vi "Izhikevich_model.vi"() -> ()   [LabVIEW 2019]
panel:
  in  "Array":dbl[](array[slide]) scale=0.0..15.0
  out "u":T1(graph)
  in  "Address Selector":i32[](array[numeric])
  out "v":T1(graph)
  in  "Neuron Type":T2(ring)
  in  "?":bool
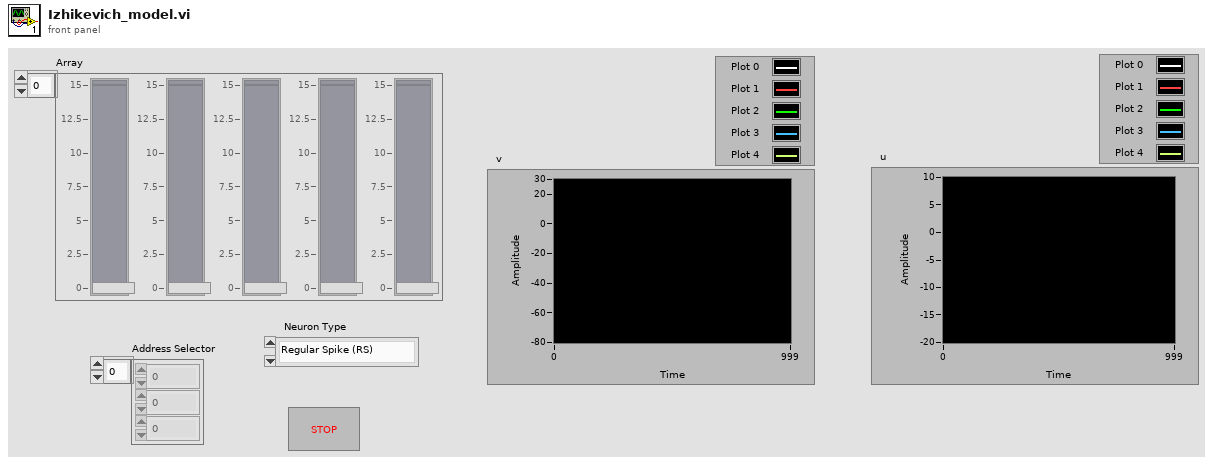
[diagram p1: front panel]
types:
  T1 = cluster{"[0]":dbl, "[1]":dbl, "[2]":dbl, "[3]":dbl, "[4]":dbl}
  T2 = enum16{"Regular Spike (RS)", "Intrinsically  Bursting (IB)", "Chattering (CH)", "Fast Spiking (FS)", "Thalamo-Cortical 1 (TC1)", "Thalamo-Cortical 2 (TC2)", "Resonator (RZ)", "Low-Threshold Spiking (LTS)", "Class 1 Excitable (C1)"}
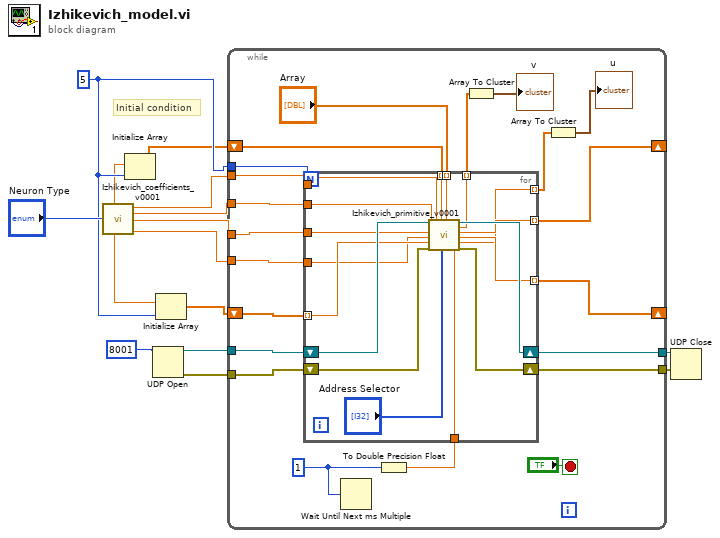
[diagram p0: block diagram]
diagram:
  w5 = 5
  # "Initial condition"
  n1 = call "Izhikevich_coefficients_v0001.vi"("Neuron Type"="Neuron Type") -> ("d"=w10:dbl, "c"=w9:dbl, "b"=w11:dbl, "a"=w12:dbl, "u0"=w4:dbl, "v0"=w3:dbl)  [unwired: 3 in]
  n2 = Initialize Array(w3, w5) -> (w2:dbl[])
  n3 = UDP Open(11:u16 8001) -> (port=w14:refnum<k16>, 0:w15:errorcluster)  [unwired: 4 in, 1 out]
  n4 = Initialize Array(w4, w5) -> (w1:dbl[])
  n5 = while {
    tunnel: w12 -> [w27]
    tunnel: w11 -> [w28]
    tunnel: w9 -> [w22]
    shift-right: [w24] -> _
    shift-left: w1 -> [w30]
    shift-right: [w25] -> _
    shift-left: w2 -> [w26]
    tunnel: w10 -> [w29]
    tunnel: w15 -> [w32]
    tunnel: w14 -> [w34]
    tunnel: [w33] -> w7
    tunnel: [w31] -> w6
    tunnel: w5 -> [w21]
    stop <- "?" stop-if-true
    w35 = u32 1 ("millisecond multiple")
    n6 = Wait Until Next ms Multiple(millisecond multiple=w35) -> ()  [unwired: 1 out]
    n7 = To Double Precision Float(number=w35) -> (double precision float=w23:dbl)
    n8 = for {
      N: w21 -> [_]
      tunnel: w30 -> [w49] mode=indexing
      tunnel: w29 -> [w48]
      tunnel: w22 -> [w47]
      tunnel: w28 -> [w46]
      tunnel: w27 -> [w45]
      tunnel: w26 -> [w44] mode=indexing
      tunnel: "Array" -> [w43] mode=indexing
      tunnel: [w42] -> w20 mode=indexing
      tunnel: [w41] -> w25 mode=indexing
      tunnel: [w40] -> w24 mode=indexing
      tunnel: [w39] -> w18 mode=indexing
      tunnel: w23 -> [w37]
      shift-right: [w52] -> w33
      shift-left: w34 -> [w53]
      shift-right: [w50] -> w31
      shift-left: w32 -> [w51]
      n9 = call "Izhikevich_primitive_v0001.vi"("UDP Network Connection in"=w53, "b"=w46, "c"=w47, "d"=w48, "u0"=w49, "error in (no error)"=w51, "a"=w45, "Numeric in"=w37, "v0"=w44, "Array"="Address Selector", "Input"=w43) -> ("UDP Network Connection out"=w52:refnum<k16>, "v"=w42:dbl, "v(t+dt)"=w41:dbl, "u(t+dt)t"=w40:dbl, "u"=w39:dbl, "error out"=w50:errorcluster)  [unwired: 3 in]
    }
    n10 = Array To Cluster(array=w20) -> (cluster=→"v":T1)
    n11 = Array To Cluster(array=w18) -> (cluster=→"u":T1)
  }
  n12 = UDP Close(connection ID=w7, 8:w6) -> ()  [unwired: 2 out]
